vi "exp1.vi"() -> ()   [LabVIEW 2022 SP3]
panel:
  out "数据记录":string[](array[string])
  out "华氏温度":dbl(knob) scale=0.0..200.0
  out "随机产生的摄氏度":dbl
  out "开氏":bool
  out "华氏":bool
  in  "停止":bool
  out "当前模式下温度值":dbl
  out "温度计":dbl(slide) scale=-20.0..400.0
  in  "模式":bool
  out "开氏温度":dbl(knob) scale=200.0..400.0
  out "电源指示灯":bool
  in  "开关":bool
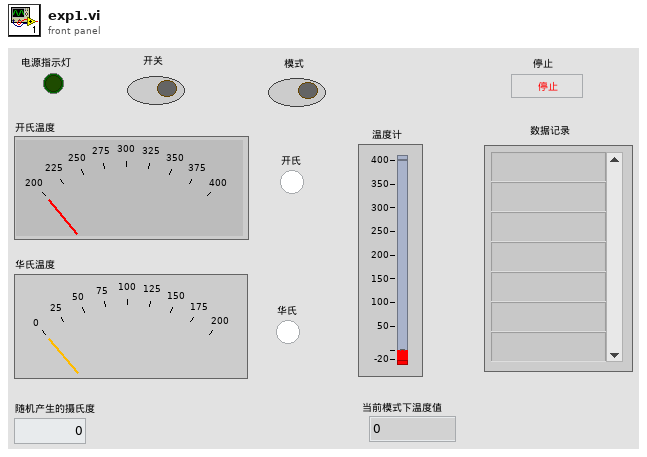
[diagram p1: front panel]
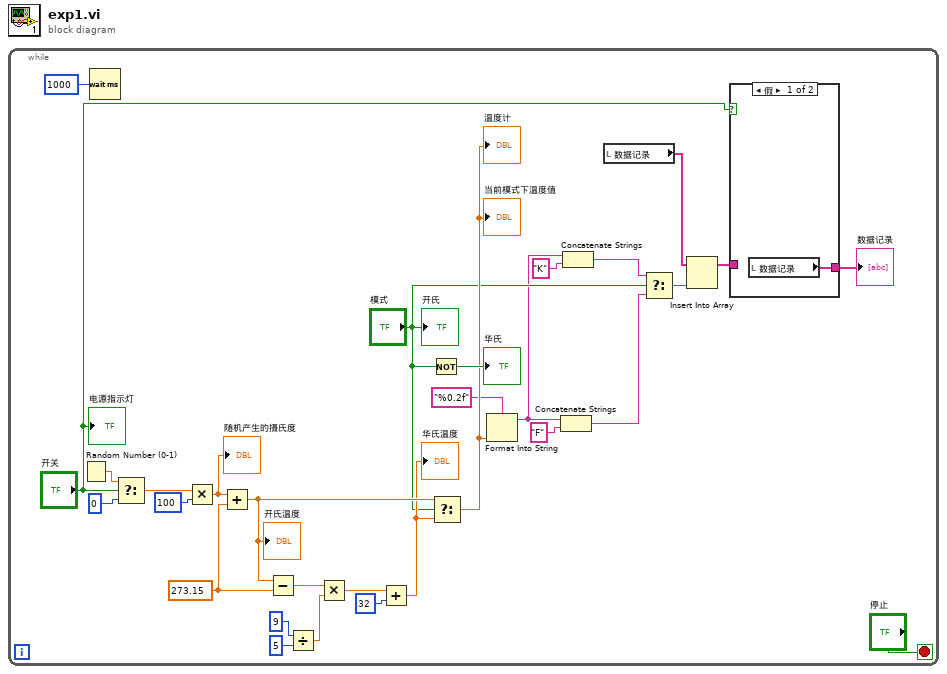
[diagram p0: block diagram]
diagram:
  n1 = while {
    stop <- "停止" stop-if-true
    w29 = 273.15
    n2 = Random Number (0-1)() -> (number: 0 to 1=w21:dbl)
    n3 = Wait (ms)(milliseconds to wait=1000) -> ()  [unwired: 1 out]
    n4 = Select(t=w21, s="开关", f=0) -> (s? t:f=w27:dbl)
    n5 = Multiply(x=w27, y=100) -> (x*y=w19:dbl)
    "随机产生的摄氏度" <- w19
    n6 = Add(x=w19, y=w29) -> (x+y=w15:dbl)
    "开氏温度" <- w15
    n7 = Subtract(x=w15, y=w29) -> (x-y=w26:dbl)
    n8 = Divide(x=9, y=5) -> (x/y=w17:dbl)
    n9 = Multiply(x=w26, y=w17) -> (x*y=w25:dbl)
    n10 = Add(x=w25, y=32) -> (x+y=w14:dbl)
    "华氏温度" <- w14
    n11 = Not(x="模式") -> (.not. x?=→"华氏":bool)
    n12 = Select(t=w15, s="模式", f=w14) -> (s? t:f=w13:dbl)
    "温度计" <- w13
    "当前模式下温度值" <- w13
    n13 = Format Into String(format string="%0.2f" ("格式字符串"), w13) -> (resulting string=w1:string)  [unwired: 2 in, 1 out]
    n14 = Concatenate Strings(w1, "F") -> (w9:string)
    n15 = Concatenate Strings(w1, "K") -> (w10:string)
    n16 = local read "数据记录"() -> (w5:string[])
    n17 = Select(t=w10, s="模式", f=w9) -> (s? t:f=w8:string)
    n18 = Insert Into Array(array=w5, new element=w8) -> (w6:string[])  [unwired: 1 in]
    n19 = case shown="假" "开关" {
      tunnel: w6 -> [_ w32]
      tunnel: [w31 w32] -> w4
      frame False {
        n20 = local read "数据记录"() -> (w31:string[])
      }
      frame True {
      }
    }
    "数据记录" <- w4
    "电源指示灯" <- "开关"
    "开氏" <- "模式"
  }
